vi "Set Async Rx.vi"(10 "Async Rx":refnum<class "Scheduler Transfer Group Bundle.lvclass">[](array[class]), 11 "Scheduler Plugin Bundle in":refnum<class "Scheduler Plugin Bundle.lvclass">) -> (3 "Scheduler Plugin Bundle out":refnum<class "Scheduler Plugin Bundle.lvclass">)   [LabVIEW 2017, in "DSF Core.lvlib" / "Scheduler Plugin Bundle.lvclass"]
uses:
  Scheduler Plugin Bundle.lvclass
  Scheduler Transfer Group Bundle.lvclass
  Scheduler Plugin Bundle.lvclass/Scheduler Plugin Bundle.ctl
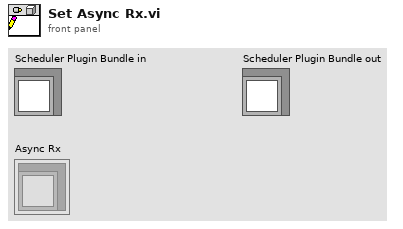
[diagram p1: front panel]
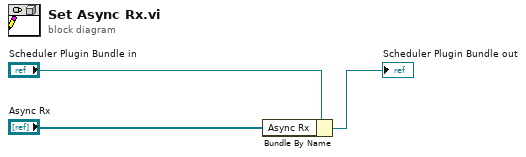
[diagram p0: block diagram]
diagram:
  n1 = Bundle By Name(cluster="Scheduler Plugin Bundle in", "Async Rx"="Async Rx") -> (→"Scheduler Plugin Bundle out":refnum<class "Scheduler Plugin Bundle.lvclass">)
